vi "medicaoIXV.vi"() -> ()   [LabVIEW 2012]
uses:
  <vilib>/Utility/file.llb/Write To Spreadsheet File (string).vi
  <vilib>/Utility/file.llb/Write To Spreadsheet File (DBL).vi
  <instrlib>/Agilent 6XXX Series/Agilent 6XXX Series.lvlib
panel:
  out "reset graph":bool=TRUE
  out "tabela":dbl[][](array[numeric])
  in  "Tab Control":enum32{"Entrada de dados", "Saída de dados"}(tab)
  in  "T.J":dbl caption="Tensão\ndo joelho"
  in  "p.a.j":dbl caption="Pontos antes\ndo joelho"
  in  "nMedições":i16=1 caption="N° medições" min=1
  in  "area":dbl caption="Área da célula"
  in  "Tipo":string caption="Tipo da célula"
  in  "Formato":u16(ring) items=[".txt", ".csv"]
  out "ON/OFF1":bool caption="ON/OFF"
  in  "p.d.j":dbl caption="Pontos depois\ndo joelho"
  in  "T.M":dbl caption="Tensão máxima"
  in  "Nome da célula":string
  in  "Local":path
  in  "Delay(ms)":dbl
  in  "Start":bool
  in  "temperatura":dbl caption="Temperatura da célula"
  in  "stopProgram":bool caption="Parar Programa"
  out "Imp":dbl
  out "Vmp":dbl
  out "Pmp":dbl
  out "Icc (A)":dbl
  out "Vca (V)":dbl
  in  "Print Screen":bool
  out "IXV":cluster{"Y":dbl[], "Y":dbl[]}[](graph)
  out "output voltage":dbl
  out "Tensao Atual (V)":dbl
  out "Corrente Atual\n(A)":dbl
  out "Ponto Atual":i32
  out "tabela":dbl[][](array[numeric]) caption="TABELA DE DADOS\nTensão(Fonte)      Pontos             Tensao           Corrente" format="%0.3f"
  in  "stop":bool caption="Parar Medição"
  out "ON/OFF2":bool caption="ON/OFF"
  in  "CorrenteGraph":dbl
  in  "TensaoGraph":dbl
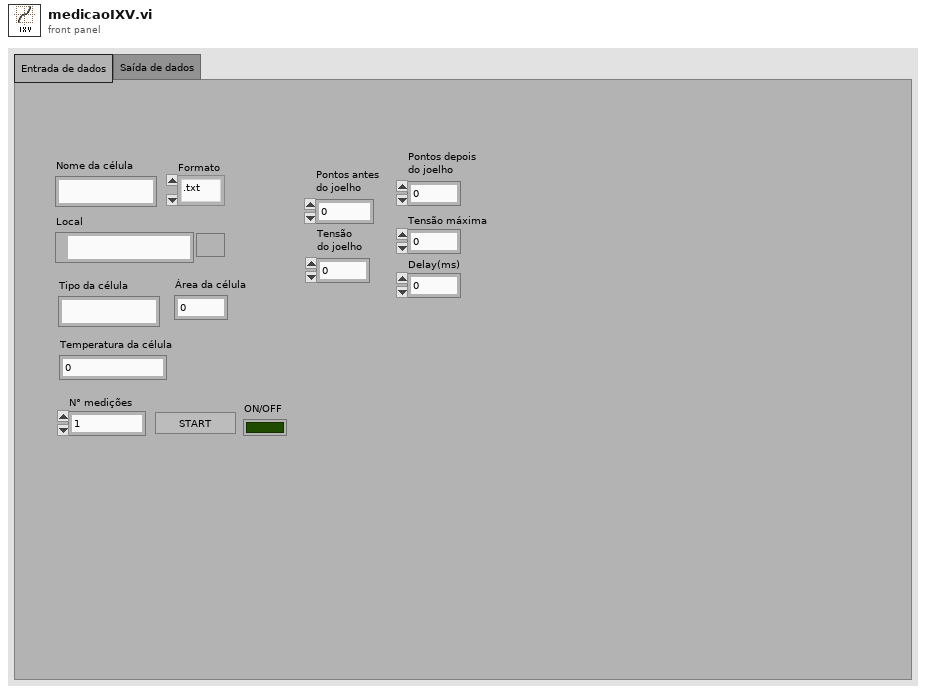
[diagram p1: front panel]
types:
  T1 = typedef "imagedata.ctl" = cluster{"image type":i32, "image depth":i32, "image":u8[], "mask":u8[], "colors":u32[], "Rectangle":cluster{"left":i16, "top":i16, "right":i16, "bottom":i16}}
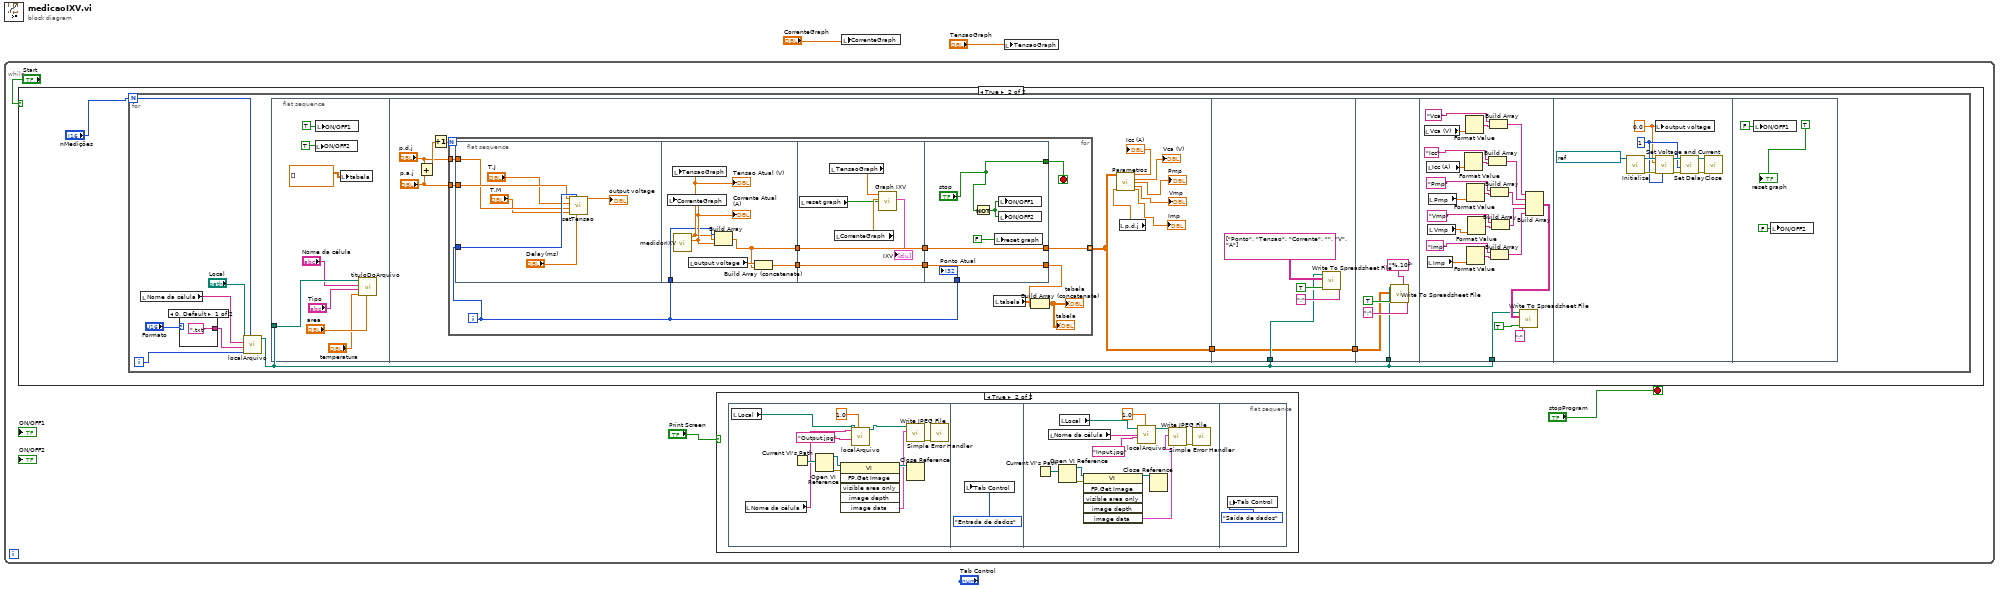
[diagram p0: block diagram]
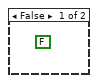
[diagram p3: hidden frame]
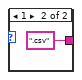
[diagram p4: hidden frame]
diagram:
  n1 = while {
    stop <- "stopProgram" stop-if-true
    n2 = case shown="True" "Start" {
      frame False {
        (unwired) FALSE
      }
      frame True {
        n3 = for {
          N: "nMedições" -> [w36]
          i -> [w32]
          n4 = local read "Nome da célula"() -> (w34:string)
          n5 = case shown="0, Default" "Formato" {
            tunnel: [".txt" ".csv"] -> w33
            frame 0, Default {
            }
            frame 1 {
            }
          }
          n6 = call "localArquivo.vi"("quantidadeDeArquivos"=w36, "numeroDoArquivo"=w32, "extensão"=w33, "Nome do arquivo"=w34, "Local"="Local") -> ("Path"=w31:path)  [unwired: 6 in]
          n7 = flat-sequence {
            tunnel: w31 -> [w49]
            tunnel: [w60] -> w39
            tunnel: w31 -> [w99]
            tunnel: [w98] -> w38
            tunnel: w39 -> [w98]
            tunnel: w31 -> [w104]
            tunnel: w38 -> [w103]
            tunnel: w31 -> [w108]
            frame #0 {
              n8 = local write "ON/OFF2"(TRUE ("ON/OFF2")) -> ()
              n9 = local write "ON/OFF1"(TRUE ("ON/OFF")) -> ()
              n10 = local write "tabela"(dbl[][] [] ("array")) -> ()
              n11 = call "tituloDoArquivo.vi"("area"="area", "temperatura"="temperatura", "Tipo"="Tipo", "Nome da célula"="Nome da célula", "file path (dialog if empty)"=w49) -> ()  [unwired: 7 in]
            }
            frame #1 {
              n12 = Add(x="p.d.j", y="p.a.j") -> (x+y=w52:dbl)
              n13 = Increment(x=w52) -> (x+1=w59:dbl)
              n14 = for {
                N: w59 -> [_]
                tunnel: [w72] -> w60 mode=indexing
                tunnel: "p.a.j" -> [w62]
                tunnel: "p.d.j" -> [w61]
                i -> [w66]
                stop <- w65 stop-if-true
                n15 = flat-sequence {
                  tunnel: w66 -> [w78]
                  tunnel: w62 -> [w76]
                  tunnel: w61 -> [w75]
                  tunnel: w66 -> [w80]
                  tunnel: [w83] -> w71
                  tunnel: [w85] -> w70
                  tunnel: [w91] -> w64
                  tunnel: [w90] -> w63
                  tunnel: w70 -> [w90]
                  tunnel: w71 -> [w91]
                  tunnel: [w96] -> w69
                  tunnel: [w97] -> w72
                  tunnel: w64 -> [w97]
                  tunnel: w63 -> [w96]
                  tunnel: w66 -> [w95]
                  tunnel: ["stop"] -> w65
                  frame #0 {
                    n16 = call "setTensao.vi"("delay(ms)"="Delay(ms)", "Ponto atual"=w78, "T.M"="T.M", "P.D.J"=w75, "T.J"="T.J", "P.A.J"=w76) -> ("output voltage"=→"output voltage":dbl)  [unwired: 5 in]
                  }
                  frame #1 {
                    n17 = call "medidorIXV.vi"() -> ("Corrente Atual"=w82:dbl, "Tensao Atual"=w81:dbl)  [unwired: 10 in]
                    "Corrente Atual\n(A)" <- w82
                    "Tensao Atual (V)" <- w81
                    n18 = local write "CorrenteGraph"(w82) -> ()
                    n19 = local write "TensaoGraph"(w81) -> ()
                    n20 = local read "output voltage"() -> (w84:dbl)
                    n21 = Build Array(w80, w81, w82) -> (w83:dbl[])
                    n22 = Build Array (concatenate)(w84, w83) -> (w85:dbl[])
                  }
                  frame #2 {
                    n23 = local read "reset graph"() -> (w86:bool)
                    n24 = local read "TensaoGraph"() -> (w89:dbl)
                    n25 = local read "CorrenteGraph"() -> (w88:dbl)
                    n26 = call "Graph IXV"("Reset"=w86, "Y Input"=w88, "X Input"=w89) -> ("XY Graph"=→"IXV":cluster{"Y":dbl[], "Y":dbl[]}[])  [unwired: 2 in, 6 out]
                  }
                  frame #3 {
                    n27 = Not(x="stop") -> (.not. x?=w93:bool)
                    n28 = local write "reset graph"(FALSE) -> ()
                    n29 = local write "ON/OFF1"(w93) -> ()
                    n30 = local write "ON/OFF2"(w93) -> ()
                    "Ponto Atual" <- w95
                  }
                }
                n31 = local read "tabela"() -> (w68:dbl[][])
                n32 = Build Array (concatenate)(w68, w69) -> (→"tabela" →"tabela":dbl[][])
              }
              n33 = local read "p.d.j"() -> (w58:dbl)
              n34 = call "Parametros.vi"("VetorDeDados"=w60, "pontos"=w58) -> ("Icc"=→"Icc (A)":dbl, "Vca"=→"Vca (V)":dbl, "Pmp"=→"Pmp":dbl, "Vmp"=→"Vmp":dbl, "Imp"=→"Imp":dbl)  [unwired: 9 in]
            }
            frame #2 {
              n35 = call-poly <vilib>:"Write To Spreadsheet File.vi"("delimiter (\\t)"=";" ("delimiter (\\t)"), "append to file? (new file:F)"=TRUE, "2D data"=string[][] [["Ponto", "Tensao", "Corrente"], ["", "V", "A"]], "file path (dialog if empty)"=w99) -> ()  [unwired: 4 in, 1 out]
            }
            frame #3 {
              n36 = call-poly <vilib>:"Write To Spreadsheet File.vi"("delimiter (\\t)"=";" ("delimiter (\\t)"), "format (%.3f)"="%.10f", "append to file? (new file:F)"=TRUE, "2D data"=w103, "file path (dialog if empty)"=w104) -> ()  [unwired: 3 in, 1 out]
            }
            frame #4 {
              n37 = local read "Vca (V)"() -> (w110:dbl)
              n38 = local read "Icc (A)"() -> (w120:dbl)
              n39 = local read "Imp"() -> (w123:dbl)
              n40 = local read "Vmp"() -> (w122:dbl)
              n41 = local read "Pmp"() -> (w121:dbl)
              n42 = Format Value(value (0)=w120) -> (output string=w113:string)  [unwired: 2 in]
              n43 = Format Value(value (0)=w110) -> (output string=w111:string)  [unwired: 2 in]
              n44 = Format Value(value (0)=w121) -> (output string=w115:string)  [unwired: 2 in]
              n45 = Format Value(value (0)=w123) -> (output string=w119:string)  [unwired: 2 in]
              n46 = Format Value(value (0)=w122) -> (output string=w117:string)  [unwired: 2 in]
              n47 = Build Array("Icc", w113) -> (w125:string[])
              n48 = Build Array("Vca", w111) -> (w124:string[])
              n49 = Build Array("Pmp", w115) -> (w126:string[])
              n50 = Build Array("Imp", w119) -> (w128:string[])
              n51 = Build Array("Vmp", w117) -> (w127:string[])
              n52 = Build Array(w124, w125, w126, w127, w128) -> (w129:string[][])
              n53 = call-poly <vilib>:"Write To Spreadsheet File.vi"("delimiter (\\t)"=";" ("delimiter (\\t)"), "append to file? (new file:F)"=TRUE, "2D data"=w129, "file path (dialog if empty)"=w108) -> ()  [unwired: 4 in, 1 out]
            }
            frame #5 {
              w132 = 0.0 ("voltage (0 V)")
              w135 = u8 1 ("channel (1)")
              n54 = call <instrlib>:"Initialize.vi"("VISA resource name"=refnum<visa-resource-name> "GPIB0::5::INSTR") -> ("error out"=w137:errorcluster, "VISA resource name out"=w136:refnum<visa-resource-name>)  [unwired: 9 in]
              n55 = local write "output voltage"(w132) -> ()
              n56 = call <instrlib>:"Set Voltage and Current.vi"("channel (1)"=w135, "error in (no error)"=w137, "voltage (0 V)"=w132, "VISA resource name"=w136) -> ("error out"=w138:errorcluster, "VISA resource name out"=w139:refnum<visa-resource-name>)  [unwired: 6 in]
              n57 = call <instrlib>:"Set Delay.vi"("error in (no error)"=w138, "channel (1)"=w135, "VISA resource name"=w139) -> ("error out"=w133:errorcluster, "VISA resource name out"=w134:refnum<visa-resource-name>)  [unwired: 7 in]
              n58 = call <instrlib>:"Close.vi"("error in (no error)"=w133, "VISA resource name"=w134) -> ()  [unwired: 9 in, 1 out]
            }
            frame #6 {
              n59 = local write "ON/OFF1"(FALSE) -> ()
              n60 = local write "ON/OFF2"(FALSE ("ON/OFF")) -> ()
              "reset graph" <- TRUE
            }
          }
        }
      }
    }
    n61 = case shown="True" "Print Screen" {
      frame False {
      }
      frame True {
        n62 = flat-sequence {
          frame #0 {
            n63 = local read "Local"() -> (w9:path)
            n64 = local read "Nome da célula"() -> (w7:string)
            n65 = Current VI's Path() -> (path=w14:path)
            n66 = Open VI Reference(vi path=w14) -> (vi reference=w15:refnum<vi>, error out=w16:errorcluster)  [unwired: 5 in]
            n67 = invoke class="VI" method="FP.Get Image"(reference=w15, error in=w16) -> (reference out=w13:refnum<vi>, "image data"=w12:T1)  [unwired: 4 in, 4 out]
            n68 = call "localArquivo.vi"("quantidadeDeArquivos"=1.0, "extensão"="Output.jpg", "Nome do arquivo"=w7, "Local"=w9) -> ("Path"=w6:path)  [unwired: 7 in]
            n69 = call <vilib>:"Write JPEG File.vi"("image data"=w12, "path to JPEG file"=w6) -> ("error out"=w11:errorcluster)  [unwired: 8 in, 1 out]
            n70 = Close Reference(reference=w13) -> ()  [unwired: 1 in, 1 out]
            n71 = call <vilib>:"Simple Error Handler.vi"("error in (no error)"=w11) -> ()  [unwired: 4 in, 5 out]
          }
          frame #1 {
            n72 = local write "Tab Control"(enum32{"Entrada de dados", "Saída de dados"}."Entrada de dados" ("Tab Control")) -> ()
          }
          frame #2 {
            n73 = Current VI's Path() -> (path=w27:path)
            n74 = local read "Nome da célula"() -> (w21:string)
            n75 = Open VI Reference(vi path=w27) -> (vi reference=w26:refnum<vi>, error out=w25:errorcluster)  [unwired: 5 in]
            n76 = local read "Local"() -> (w20:path)
            n77 = invoke class="VI" method="FP.Get Image"(reference=w26, error in=w25) -> (reference out=w28:refnum<vi>, "image data"=w23:T1)  [unwired: 4 in, 4 out]
            n78 = call "localArquivo.vi"("quantidadeDeArquivos"=1.0, "extensão"="Input.jpg", "Nome do arquivo"=w21, "Local"=w20) -> ("Path"=w19:path)  [unwired: 7 in]
            n79 = Close Reference(reference=w28) -> ()  [unwired: 1 in, 1 out]
            n80 = call <vilib>:"Write JPEG File.vi"("image data"=w23, "path to JPEG file"=w19) -> ("error out"=w24:errorcluster)  [unwired: 8 in, 1 out]
            n81 = call <vilib>:"Simple Error Handler.vi"("error in (no error)"=w24) -> ()  [unwired: 4 in, 5 out]
          }
          frame #3 {
            n82 = local write "Tab Control"(enum32{"Entrada de dados", "Saída de dados"}."Saída de dados" ("Tab Control")) -> ()
          }
        }
      }
    }
  }
  n83 = local write "CorrenteGraph"("CorrenteGraph") -> ()
  n84 = local write "TensaoGraph"("TensaoGraph") -> ()
